vi "KH TURCK ETHERNETIP IOL Events.vi"(8 "Data_IO":T2, 11 "DataItem.Data":u8[](array[numeric])) -> (3 "Events":T1)   [LabVIEW 2021]
uses:
  KH TURCK ETHERNETIP TDef Enum IOL Data.ctl
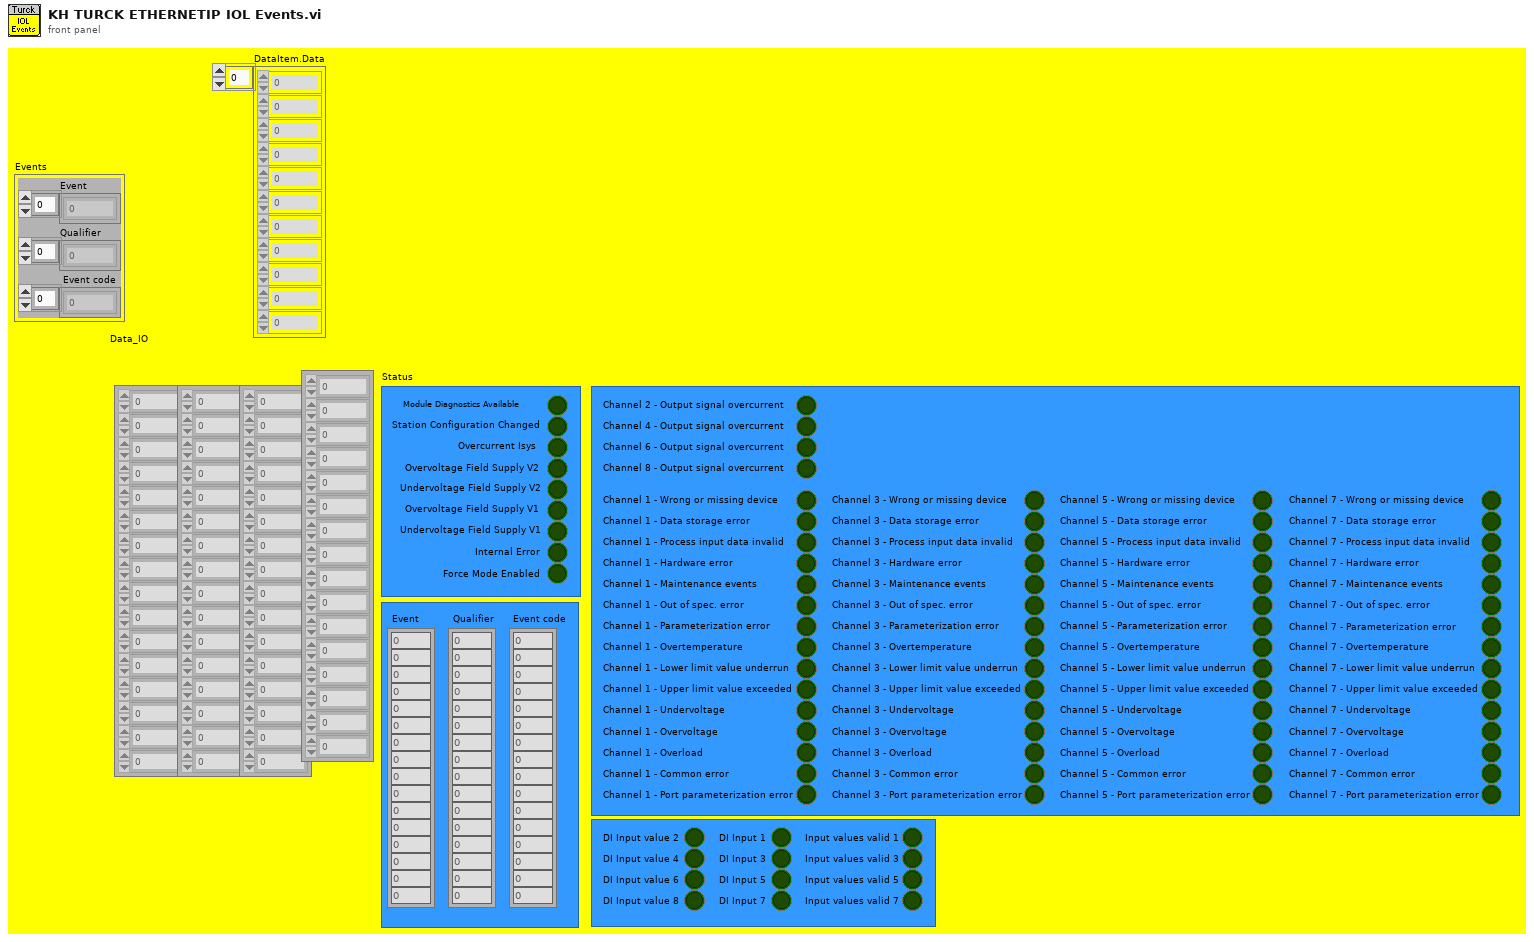
[diagram p1: front panel]
types:
  T1 = cluster{"Event":u8[], "Qualifier":u8[], " Event code":u16[]}
  T2 = typedef "KH TURCK ETHERNETIP TDef Enum IOL Data.ctl" = cluster{"Data_Port1":u16[], "Data_Port3":u16[], "Data_Port5":u16[], "Data_Port7":u16[], "Status":cluster{"Undervoltage Field Supply V2":bool, "Overvoltage Field Supply V1":bool, "Undervoltage Field Supply V1":bool, "Internal Error":bool, "Module Diagnostics Available":bool, "Station Configuration Changed":bool, "Overcurrent Isys":bool, "Overvoltage Field Supply V2":bool, "Force Mode Enabled":bool}, "Diagnostics":cluster{"Channel 2 - Output signal overcurrent":bool, "Channel 4 - Output signal overcurrent":bool, "Channel 6 - Output signal overcurrent":bool, "Channel 8 - Output signal overcurrent":bool, "Channel 1 - Wrong or missing device":bool, "Channel 3 - Wrong or missing device":bool, "Channel 5 - Wrong or missing device":bool, "Channel 7 - Wrong or missing device":bool, "Channel 1 - Data storage error":bool, "Channel 3 - Data storage error":bool, "Channel 5 - Data storage error":bool, "Channel 7 - Data storage error":bool, "Channel 1 - Process input data invalid":bool, "Channel 3 - Process input data invalid":bool, "Channel 5 - Process input data invalid":bool, "Channel 7 - Process input data invalid":bool, "Channel 1 - Hardware error":bool, "Channel 3 - Hardware error":bool, "Channel 5 - Hardware error":bool, "Channel 7 - Hardware error":bool, "Channel 1 - Maintenance events":bool, "Channel 3 - Maintenance events":bool, "Channel 5 - Maintenance events":bool, "Channel 7 - Maintenance events":bool, "Channel 1 - Out of spec. error":bool, "Channel 3 - Out of spec. error":bool, "Channel 5 - Out of spec. error":bool, "Channel 7 - Out of spec. error":bool, "Channel 1 - Parameterization error":bool, "Channel 3 - Parameterization error":bool, "Channel 5 - Parameterization error":bool, "Channel 1 - Overtemperature":bool, "Channel 3 - Overtemperature":bool, "Channel 5 - Overtemperature":bool, "Channel 7 - Overtemperature":bool, "Channel 1 - Lower limit value underrun":bool, "Channel 3 - Lower limit value underrun":bool, "Channel 5 - Lower limit value underrun":bool, "Channel 7 - Lower limit value underrun":bool, "Channel 1 - Upper limit value exceeded":bool, "Channel 3 - Upper limit value exceeded":bool, "Channel 5 - Upper limit value exceeded":bool, "Channel 7 - Upper limit value exceeded":bool, "Channel 1 - Undervoltage":bool, "Channel 3 - Undervoltage":bool, "Channel 5 - Undervoltage":bool, "Channel 7 - Undervoltage":bool, "Channel 1 - Overvoltage":bool, "Channel 3 - Overvoltage":bool, "Channel 5 - Overvoltage":bool, "Channel 7 - Overvoltage":bool, "Channel 1 - Overload":bool, "Channel 3 - Overload":bool, "Channel 5 - Overload":bool, "Channel 7 - Overload":bool, "Channel 1 - Common error":bool, "Channel 3 - Common error":bool, "Channel 5 - Common error":bool, "Channel 7 - Common error":bool, "Channel 1 - Port parameterization error":bool, "Channel 3 - Port parameterization error":bool, "Channel 5 - Port parameterization error":bool, "Channel 7 - Parameterization error":bool, "Channel 7 - Port parameterization error":bool}, "Events":cluster{"Event":u8[], "Qualifier":u8[], " Event code":u16[]}, "DXP":cluster{"DI Input value 2":bool, "DI Input value 4":bool, "DI Input value 6":bool, "DI Input value 8":bool, "DI Input 1":bool, "DI Input 3":bool, "DI Input 5":bool, "DI Input 7":bool, "Input values valid 1":bool, "Input values valid 3":bool, "Input values valid 5":bool, "Input values valid 7":bool}}
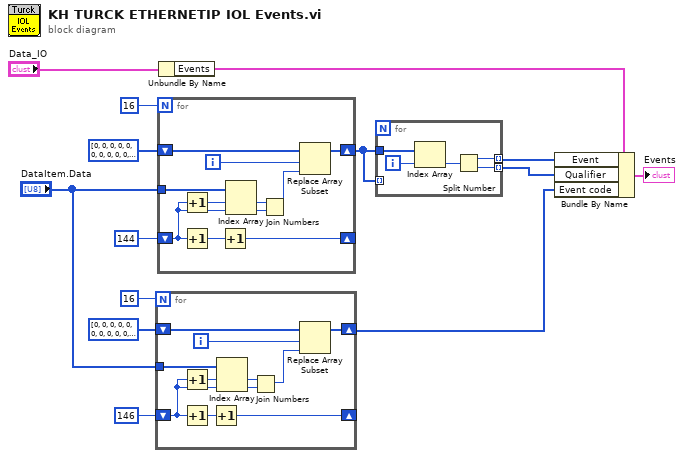
[diagram p0: block diagram]
diagram:
  n1 = for {
    N: 16 -> [_]
    shift-right: [w24] -> w3
    shift-left: u16[] [0, 0, 0, 0, 0, 0, 0, 0, 0, 0, 0, 0, 0, 0, 0, 0] ("DataItem.Data 2") -> [w25]
    tunnel: "DataItem.Data" -> [w23]
    shift-right: [w16] -> _
    shift-left: 146 ("index") -> [w15]
    i -> [w19]
    n2 = Increment(x=w15) -> (x+1=w22:i32)
    n3 = Increment(x=w15) -> (x+1=w17:i32)
    n4 = Increment(x=w17) -> (x+1=w16:i32)
    n5 = Index Array(array=w23, index #1=w22, index #2=w15) -> (element #1=w21:u8, element #2=w20:u8)
    n6 = Join Numbers(hi=w21, lo=w20) -> ((hi.lo)=w18:u16)
    n7 = Replace Array Subset(array=w25, new element=w18, index=w19) -> (w24:u16[])
  }
  n8 = for {
    N: 16 -> [_]
    shift-right: [w35] -> w1
    shift-left: u16[] [0, 0, 0, 0, 0, 0, 0, 0, 0, 0, 0, 0, 0, 0, 0, 0] ("DataItem.Data 2") -> [w36]
    tunnel: "DataItem.Data" -> [w34]
    shift-right: [w27] -> _
    shift-left: 144 ("index") -> [w26]
    i -> [w30]
    n9 = Increment(x=w26) -> (x+1=w33:i32)
    n10 = Increment(x=w26) -> (x+1=w28:i32)
    n11 = Increment(x=w28) -> (x+1=w27:i32)
    n12 = Index Array(array=w34, index #1=w33, index #2=w26) -> (element #1=w32:u8, element #2=w31:u8)
    n13 = Join Numbers(hi=w32, lo=w31) -> ((hi.lo)=w29:u16)
    n14 = Replace Array Subset(array=w36, new element=w29, index=w30) -> (w35:u16[])
  }
  n15 = Unbundle By Name("Data_IO") -> ("Events"=w13:T1)
  n16 = for {
    tunnel: w1 -> [w41]
    tunnel: [w38] -> w10 mode=indexing
    tunnel: [w37] -> w4 mode=indexing
    tunnel: w1 -> [_] mode=indexing
    i -> [w39]
    n17 = Index Array(array=w41, index=w39) -> (element=w40:u16)
    n18 = Split Number(x=w40) -> (hi(x)=w38:u8, lo(x)=w37:u8)
  }
  n19 = Bundle By Name(cluster=w13, "Event"=w10, "Qualifier"=w4, "Event code"=w3) -> (→"Events":T1)
